vi "flipflop.vi"(8 "Overide false":bool, 9 "Overide true":bool, 10 "Start value":bool, 11 "flip":bool) -> (3 "flop":bool)   [LabVIEW 2015]
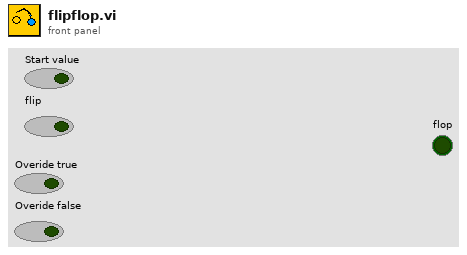
[diagram p1: front panel]
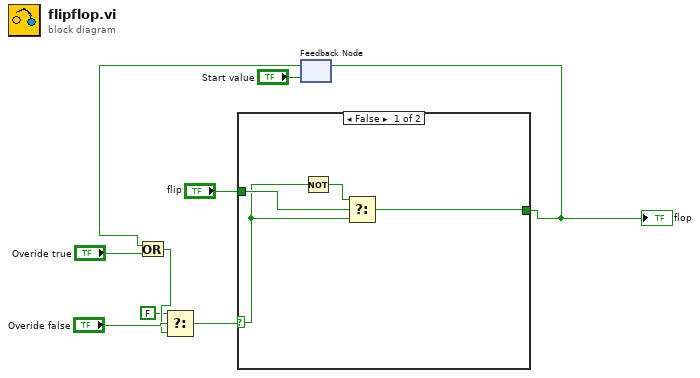
[diagram p0: block diagram]
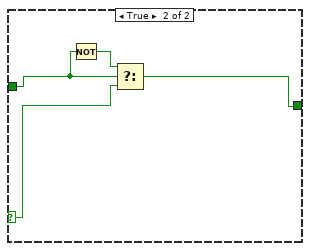
[diagram p2: hidden frame]
diagram:
  n1 = feedback #1("Start value") -> (w6:bool)
  n2 = Or(x=w6, y="Overide true") -> (x .or. y?=w2:bool)
  n3 = Select(t=FALSE, s="Overide false", f=w2) -> (s? t:f=w4:bool)
  n4 = case shown="False" w4 {
    selector: w4 -> [w11 w17]
    tunnel: "flip" -> [w12 w15]
    tunnel: [w10 w14] -> w8
    frame False {
      n5 = Not(x=w11) -> (.not. x?=w13:bool)
      n6 = Select(t=w13, s=w12, f=w11) -> (s? t:f=w10:bool)
    }
    frame True {
      n7 = Not(x=w15) -> (.not. x?=w16:bool)
      n8 = Select(t=w16, s=w15, f=w17) -> (s? t:f=w14:bool)
    }
  }
  "flop" <- w8
  n9 = feedback-in #1(w8) -> ()
